vi "Launcher.vi"   [LabVIEW 2019]
uses:
  DT Controller/DT Controller/DT Controller.lvclass
  C:/Program Files/National Instruments/LabVIEW 2019/vi.lib/ActorFramework/Actor/Actor.lvclass
  <vilib>/ActorFramework/Actor/Actor.lvclass
panel:
  # "Launch DeepTrainer"
types:
  T1 = enum32{"Invalid", "Standard", "Closed", "Hidden", "Minimized", "Maximized"}
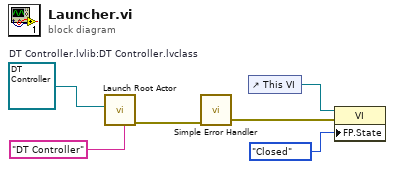
[diagram p0: block diagram]
diagram:
  w6 = refnum<class "DT Controller.lvclass"> refnum  # DT Controller.lvlib:DT Controller.lvclass
  n1 = call <vilib>:"Launch Root Actor.vi"("Debug Alias"="DT Controller", "Actor"=w6) -> ("error out"=w5:errorcluster)  [unwired: 8 in, 1 out]
  n2 = call <vilib>:"Simple Error Handler.vi"("error in (no error)"=w5) -> ("error out"=w4:errorcluster)  [unwired: 4 in, 4 out]
  n3 = control-ref of="This VI"() -> (w1:refnum<vi>)
  n4 = property class="VI"(reference=w1, error in=w4, "FP.State"=T1."Closed" ("Front Panel Window:State")) -> ()  [unwired: 2 out]
